vi "Write General Settings.vi"(8 "error in (no error)":errorcluster, 10 "General Settings":T1, 11 "IP_Communication in":refnum<class "IP_Communication.lvclass">) -> (0 "error out":errorcluster, 3 "IP_Communication out":refnum<class "IP_Communication.lvclass">)   [LabVIEW 2020, in "Communication Classes.lvlib" / "IP_Communication.lvclass"]
uses:
  IP_Communication.lvclass
  typedefs/Endpoint Tag.ctl
  typedefs/General Settings.ctl
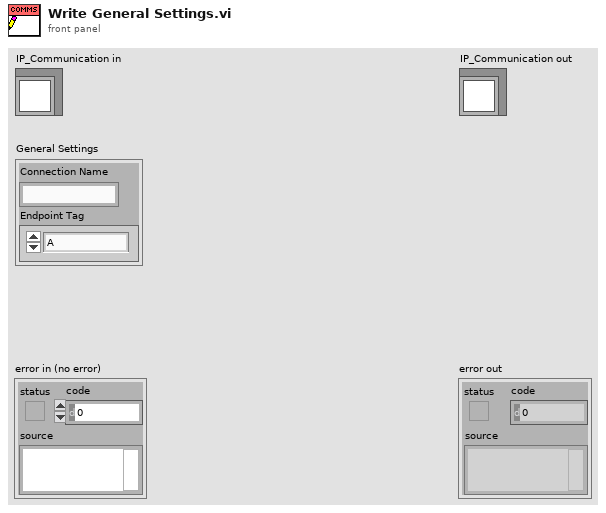
[diagram p1: front panel]
types:
  T1 = typedef "Communication Classes.lvlib/IP_Communication.lvclass/General Settings.ctl" = cluster{"Connection Name":string, "Endpoint Tag":T2}
  T2 = typedef "Communication Classes.lvlib/IP_Communication.lvclass/Endpoint Tag.ctl" = enum8{"A", "B"}
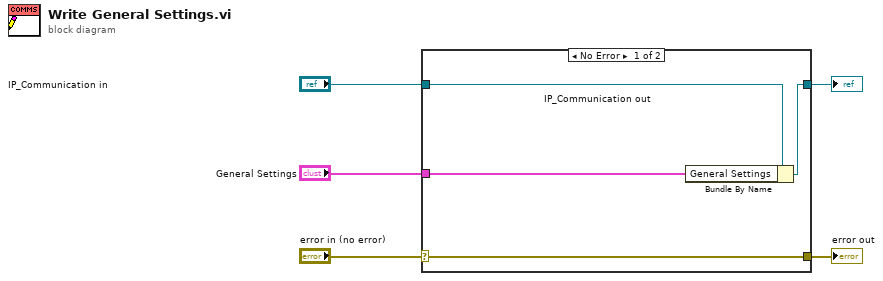
[diagram p0: block diagram]
diagram:
  n1 = case shown="No Error" "error in (no error)" {
    selector: "error in (no error)" -> [w9 w10]
    tunnel: [w9 w10] -> w4
    tunnel: [w7 w11] -> w2
    tunnel: "IP_Communication in" -> [w8 w11]
    tunnel: "General Settings" -> [w6 _]
    frame No Error {
      n2 = Bundle By Name(cluster=w8, "General Settings"=w6) -> (w7:refnum<class "IP_Communication.lvclass">)
    }
    frame Error {
    }
  }
  "error out" <- w4
  "IP_Communication out" <- w2
